vi "Untitled 2.vi"() -> ()   [LabVIEW 2019]
uses:
  TypeDef/GUI Alarm Lelel 4 points.ctl
  TypeDef/GUI Alarm Level one point.ctl
panel:
  in  "?":cluster{"HIHI":T1, "HI":T1}
  in  "?":T2
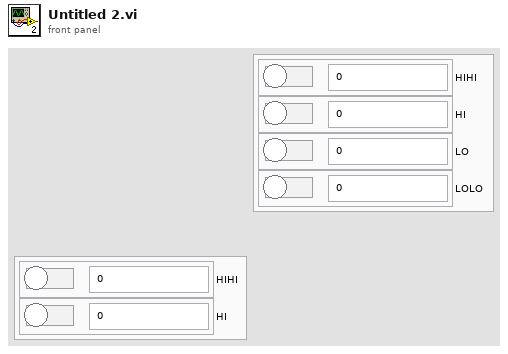
[diagram p1: front panel]
types:
  T1 = typedef "GUI Alarm Level one point.ctl" = cluster{"EN":bool, "VAL":dbl}
  T2 = typedef "GUI Alarm Lelel 4 points.ctl" = cluster{"HIHI":T1, "HI":T1, "LO":T1, "LOLO":T1}
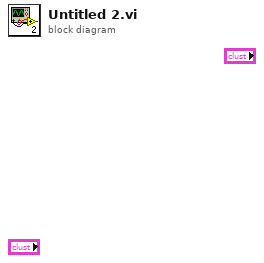
[diagram p0: block diagram]
diagram:
